vi "prepare16 v3.vi"(0 "db":dbl, 1 "ppStmt":dbl, 5 "zSql":u32, 7 "nByte":i32, 9 "prepFlags":u32, 11 "error in (no error)":errorcluster, 12 "pzTail":u32) -> (3 "ppStmt out":dbl, 4 "db out":dbl, 6 "function return":i32, 15 "error out":errorcluster)   [LabVIEW 2020, in "sqlite3.lvlib"]
uses:
  sqlite3.lvlib
  errstr.vi
  bin/sqlite3_64.dll
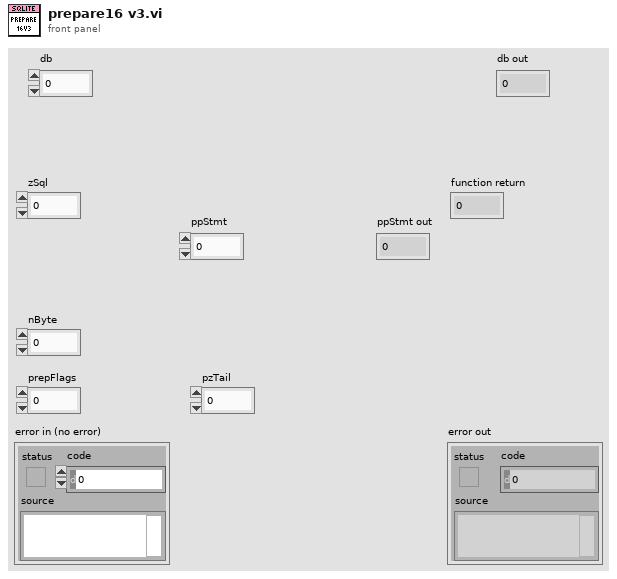
[diagram p1: front panel]
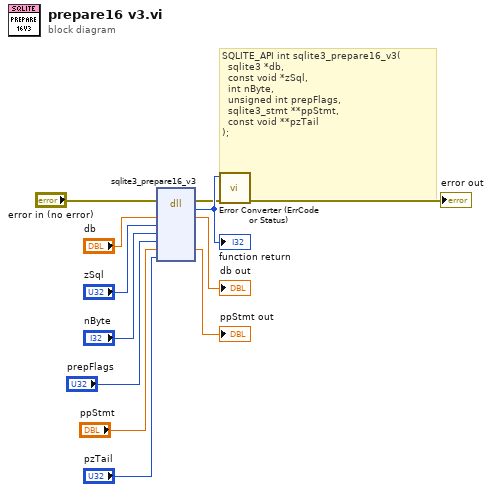
[diagram p0: block diagram]
diagram:
  # "SQLITE_API int sqlite3_prepare16_v3(\n  sqlite3 *db,            \n  const void *zSql,       \n  int nByte,              \n  unsigned int prepFlags, \n  sqlite3_stmt **ppStmt,  \n  const void **pzTail     \n);"
  n1 = dll-call lib="D:/Project/Labview-Projects/database-configuration/externals/sqlite3/Source/bin/sqlite3_*.*" fn="sqlite3_prepare16_v3"(error in="error in (no error)", "db"="db", "zSql"="zSql", "nByte"="nByte", "prepFlags"="prepFlags", "ppStmt"="ppStmt", "pzTail"="pzTail") -> (error out=w2:errorcluster, w12:i32, "db"=→"db out":dbl, "ppStmt"=→"ppStmt out":dbl)  [unwired: 6 in, 1 out]
  "function return" <- w12
  n2 = call "Error Converter (ErrCode or Status).vi"("error in (no error)"=w2, "error code"=w12) -> ("error out"=→"error out":errorcluster)  [unwired: 9 in]
